vi "GUI_HTT_CTRLv5.vi"() -> ()   [LabVIEW 2020]
uses:
  Shared/GUI_Template/GUI_master/tcp_new_data_event.ctl
  Shared/GUI_Template/GUI_master/tcp new data cluster.ctl
  GUI_TestStand/Fire button.ctl
  <vilib>/Utility/config.llb/Write Key (I32).vi
  <vilib>/Utility/config.llb/Write Key (String).vi
  <vilib>/Platform/browser.llb/Open URL in Default Browser (string).vi
  <vilib>/Utility/config.llb/NI_LVConfig.lvlib
panel:
  out "Opening Time High Value":dbl
  in  "GUIdevice 18":string="HTT-DG645_6_B"
  in  "GUIdevice 17":string="HTT-ManualParameterBool"
  in  "MagSpecGUI 2":bool caption="PicoL GUI"
  out "Delay.Ch C::16":dbl caption="Lamp Timing (680 us is max.)" min=-1.0 max=1.0 format="%#_6e"
  in  "GUIdevice 16":string="HTT-DG645_5Hz"
  in  "AJG Builds":bool caption="PicoB GUI"
  in  "HTW Wiki":bool caption="Google Drive"
  in  "GEECS Website":bool caption="Google Drive"
  in  "HELP":bool caption="Google Drive"
  in  "GUIdevice 15":string="HTT-NewportXPS"
  in  "OK Button":bool
  in  "Date":string="0"
  in  "Create Log":bool caption="LogTable"
  in  "Scan":T1(ring)
  out "standard output":string
  in  "LogEpilog":bool caption="LogTable"
  in  "New day new log":bool=TRUE
  in  "LogTable":bool
  in  "PicoL2":bool caption="PicoL GUI"
  in  "1Wire B GUI":bool caption="PicoL GUI"
  out "fire::12":string="fire" caption="fire"
  in  "Wavelength.Channel0::14":enum16{"248", "355", "532", "800", "2940"}(ring)=enum."532"
  in  "Wavelength.Channel1::14":enum16{"248", "355", "532", "800", "2940"}(ring)=enum."800"
  in  "Wavelength.Channel0::13":enum16{"532", "800"}(ring)=enum."800"
  in  "EnergyRange.Channel0::14":T2(ring)=enum."400mJ"
  in  "EnergyRange.Channel1::14":T2(ring)=enum."400mJ"
  in  "EnergyRange.Channel0::13":T3(ring)=enum."200mJ"
  in  "energy.channel 1::14":dbl caption="Energy Gaia" min=0.0 max=200.0 format="%#_13g"
  out "Energy (J)":dbl
  in  "Multiplicator":dbl=15.3
  in  "GUIdevice 14":string="HTT-Energy-S-G"
  in  "Calibration X":dbl=66.6
  in  "Multiplicator Scatter":dbl=100.0
  out "Energy Scatter (J)":dbl
  out "Energy (J)":dbl
  in  "energy.channel 0::13":dbl caption="Energy Drive" min=0.0 max=10.0 format="%#_13g"
  in  "energy.channel 0::14":dbl caption="Energy Scatter" min=0.0 max=20.0 format="%#_13g"
  in  "GUIdevice 13":string="HTT-Energy-D"
  in  "IR Pt Exp And Comp":bool caption="PicoL GUI"
  in  "Position.Axis 2::10":dbl caption="y/vert." min=-6000.0 max=6000.0
  in  "Position.Axis 3::10":dbl caption="Scatter Mode z" min=-100.0 max=100.0
  in  "Position.Axis 1::10":dbl caption="x/hor." min=-150.0 max=150.0
  in  "Position.Axis 2::11":dbl caption="Translation" min=-50.0 max=50.0
  in  "Position.Axis 3::11":dbl caption="Rotation G1" min=-360.0 max=360.0
  in  "Position.Axis 1::11":dbl caption="Rotation G2" min=-360.0 max=360.0
  in  "Ethernet Powerstrip":bool caption="Google Drive"
  in  "Position.Axis 3::4":dbl caption="z" min=-20.0 max=26.0
  in  "Position.Axis 1::15":dbl caption="Delay Stage" min=-600.0 max=600.0
  in  "FilterWheelB1":bool caption="PicoB GUI"
  in  "Search Log":bool caption="PicoL GUI"
  in  "Experiment \n(if, shadow, topjet)":bool caption="PicoL GUI"
  in  "RemoteDesktop":bool caption="PicoL GUI"
  in  "Experiment \n(e-profile, xrays)":bool caption="PicoL GUI"
  in  "IR TC Pointing (17s)":bool caption="PicoL GUI"
  in  "Scatter Depletion":bool caption="PicoL GUI"
  in  "Scatter IR Amps":bool caption="PicoL GUI"
  in  "Drive TC Pt":bool caption="PicoL GUI"
  in  "Gaia Profiles":bool caption="PicoL GUI"
  in  "Gaia Pointing":bool caption="PicoL GUI"
  in  "IR Exp and Comp":bool caption="PicoL GUI"
  in  "HTT Interactive":bool caption="PicoL GUI"
  in  "GUIdevice 12":string="HTT-DG645"
  in  "Delay.Ch C::12":dbl caption="Delay" min=-0.1 max=2.0 format="%#_6e"
  in  "Delay.Ch D::12":dbl caption="Width" min=-0.1 max=2.0 format="%#_6e"
  in  "Amplitude.Ch CD::12":dbl caption="DG645" min=0.5 max=5.0
  in  "Field::1":dbl caption="B-Field" min=0.0 max=10000.0
  in  "Delay.Ch A::18":dbl caption="Delay" min=0.0 max=1.0 format="%#_6e"
  in  "Delay.Ch B::18":dbl caption="Width" min=0.0 max=1.0 format="%#_6e"
  in  "Amplitude.Ch AB::18":dbl caption="Cam Trig Amp" min=0.5 max=5.0
  in  "1Wire L GUI":bool caption="PicoL GUI"
  in  "Opt. Spectrometer":bool caption="PicoL GUI"
  in  "SingleCamGUI":bool caption="PicoL GUI"
  in  "Exp Editor":bool caption="PicoL GUI"
  in  "DB Editor":bool caption="PicoL GUI"
  in  "Laser Log":bool caption="PicoL GUI"
  in  "LoasisNetDropSchedule":bool caption="PicoL GUI"
  in  "LVStarter":bool caption="PicoL GUI"
  in  "MasterControl":bool caption="PicoL GUI"
  in  "MagSpecGUI":bool caption="PicoL GUI"
  in  "HTT Daily Ops Google Folder":bool caption="Google Drive"
  in  "Depletion Cams":bool caption="PicoL GUI"
  in  "D-L-Cams":bool caption="PicoL GUI"
  in  "Position.Axis 2::5":dbl caption="Mode Out z" min=0.0 max=150.0
  in  "Position.Axis 1::4":dbl caption="Blade" min=-25.0 max=25.0
  in  "Amplitude.Ch CD::18":dbl caption="Trigger Amplitude (V)" min=0.5 max=5.0
  in  "Position.Axis 3::5":dbl caption="Drive Mode In z" min=0.0 max=150.0
  in  "Position.Axis 1::5":dbl caption="Mode Out Wedge" min=0.0 max=25.0
  out "Position.Axis3::2":dbl caption="Rotation G1" min=-180.0 max=180.0 format="%#_13g"
  out "Position.Axis2::2":dbl caption="Rotation G2" min=-180.0 max=180.0 format="%#_13g"
  in  "Position.Axis1::2":dbl caption="Translation" min=-60000.0 max=60000.0 format="%#_13g"
  in  "PicoL":bool caption="PicoL GUI"
  in  "PicoB":bool caption="PicoB GUI"
  in  "AnalogOutput.Channel 0::9":dbl caption="Pressure Ctrl (V)" min=0.0 max=10.0
  in  "Delay.Ch D::18":dbl caption="Opening time (s)" min=0.0 max=100000000000.0 format="%#_6e"
  in  "value1::17":bool caption="Jet Enable"
  in  "value0::17":bool caption="Jet Trigger"
  in  "Position.Axis 3::3":dbl caption="Jet Z" min=0.0 max=25.0
  in  "Position.Axis 2::3":dbl caption="Jet Y" min=11.8 max=25.0
  in  "Position.Axis 1::3":dbl caption="Jet X" min=0.0 max=25.0
  in  "Position.Axis 3::6":dbl caption="Probe delay" min=0.0 max=200.0
  in  "GUIdevice 11":string="HTT-ESP05"
  in  "GUIdevice 8":string="HTT-BNC"
  in  "GUIdevice 6":string="HTT-ESP04"
  in  "GUIdevice 5":string="HTT-ESP03"
  in  "Fire Button":T4=TRUE
  out "error IO 2":errorcluster
  out "fire::10":string
  out "tcp data event":T5
  in  "UDP error message":string
  in  "GUIdevice 7":string="HTT-Pulsar"
  in  "GUIdevice 2":string="HTT-Aerotech"
  in  "GUIdevice 10":string="HTT-ESP06"
  in  "GUIdevice 4":string="HTT-ESP02"
  in  "GUIdevice 1":string="HTT-MagTeslameter-DTM141"
  in  "GUIdevice 3":string="HTT-ESP01"
  in  "GUIdevice 9":string="HTT-HighPressureDAQ"
  in  "Delay.Ch C::18":dbl caption="Jet timing (s)" min=0.0 max=100.0 format="%#_6f"
  in  "stop":bool
  # "Energy"
  # "CAP"
  # "HTT CONTROL CENTER"
  # "Drive"
  # "Gas Jet"
  # "GUI Collection"
  # "Compressor"
  # "Drive Cameras"
  # "Mode Imager"
  # "Probe Delay Line"
  # "Scatter Cameras"
  # "Scatter"
  # "Compressor"
  # "Electronics"
  # "DG645_6_B"
  # "Mode Imager"
  # "Experiment GUIs"
  # "Scatter Delay vs. Drive"
  # "Turning Mirror"
  # "MC Links"
  # "Docu"
  # "Log Maker"
  # "Energy"
  # "yyyy, mm, dd"
  # "Adjustment GUIs"
  # "Drive"
  # "Drive Comp."
  # "Scatter"
  # "Range"
  # "Wavelength"
  # "v0.7   04/16/2021"
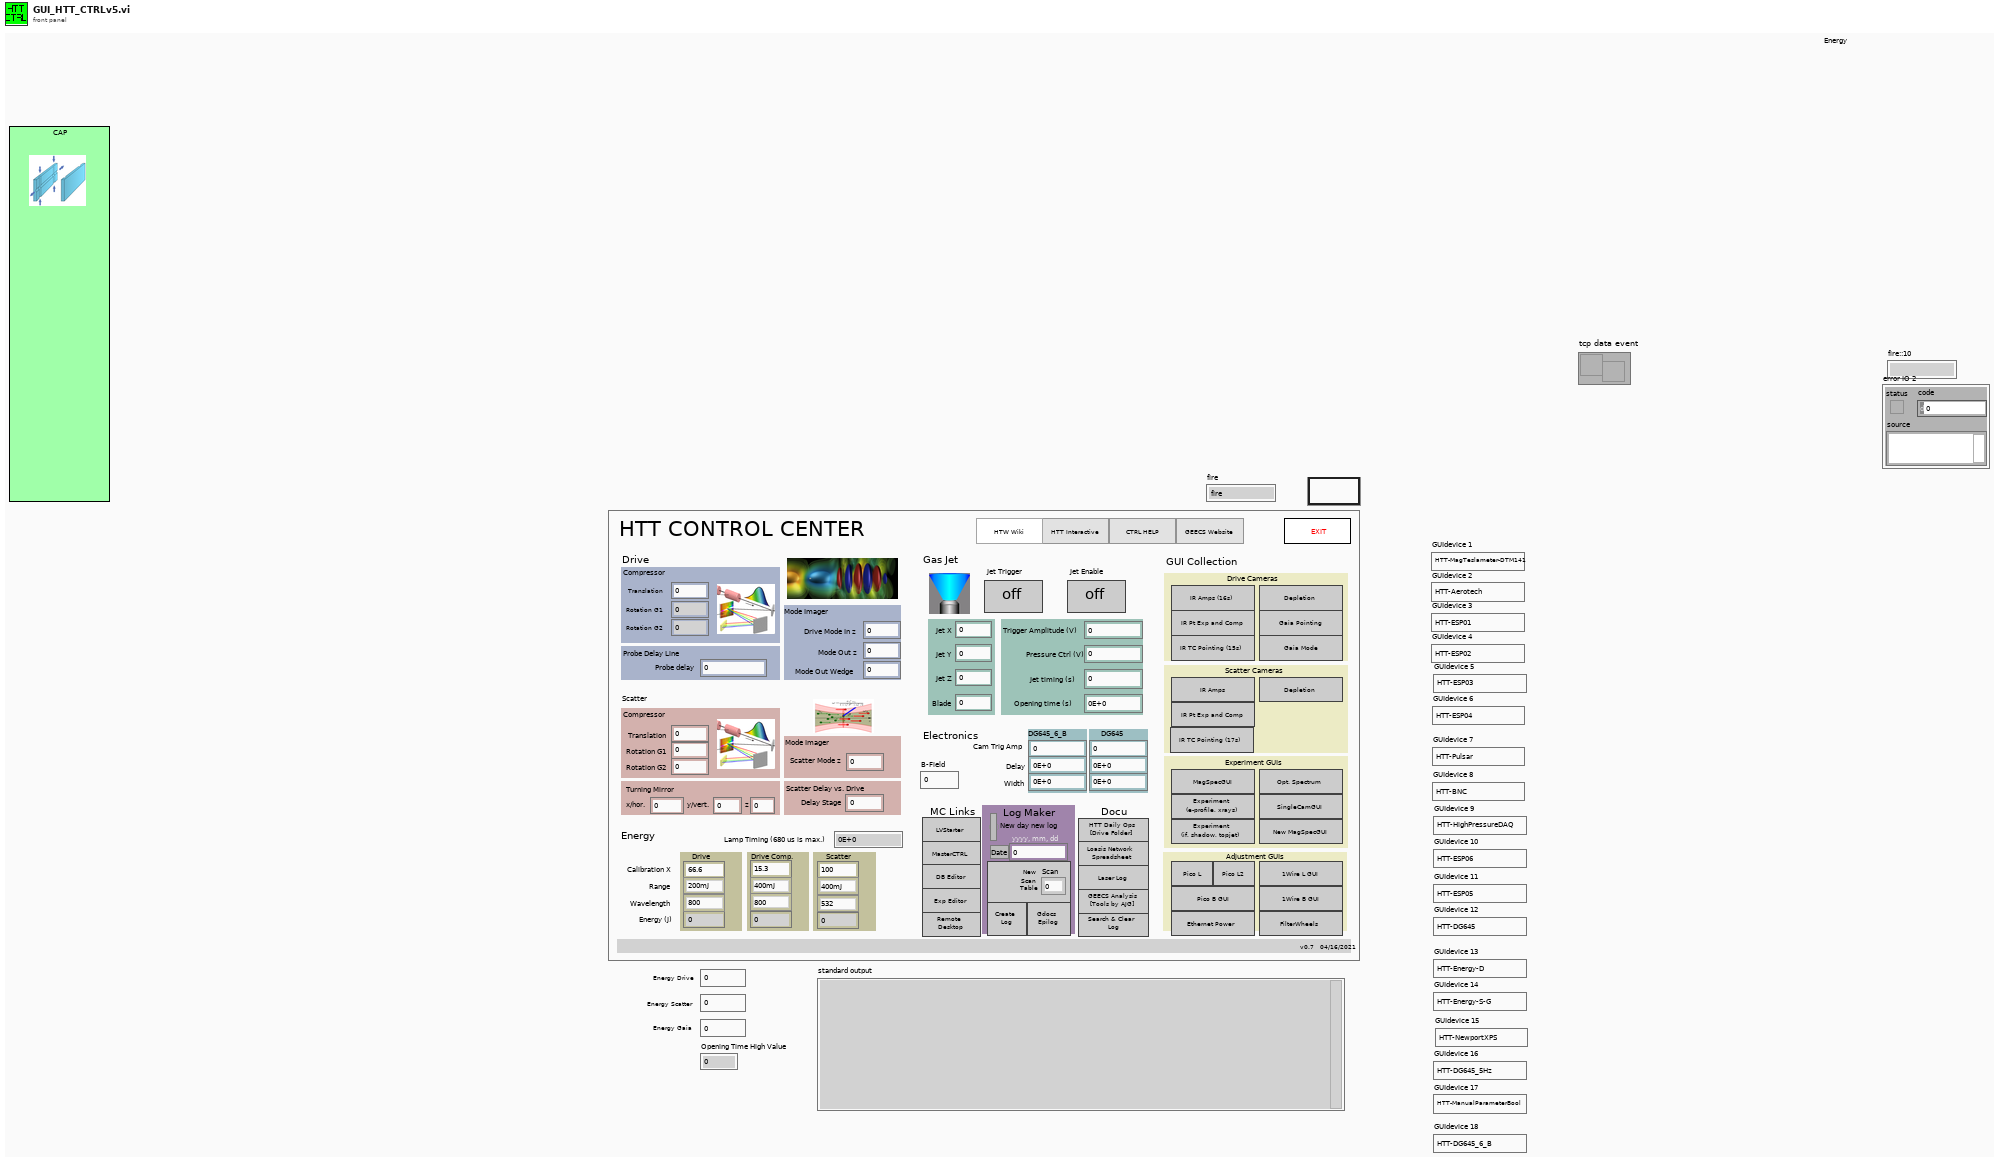
[diagram p1: front panel]
types:
  T1 = enum16{"0", "1", "2", "3", "4", "5", "6", "7", "8", "9", "10", "11", "12", "13", "14", "15", "16", "17", "18", "19", "20", "21", "22", "23", "24", "25", "26", "27", "28", "29", "30", "31", "32", "33", "34", "35", "36", "37", "38", "39", "40", "41", "42", "43", "44", "45", "46", "47", "48", "49", "50", "51", "52", "53", "54", "55", "56", "57", "58", "59", "60", "61", "62", "63", "64", "65", "66", "67", "68", "69", "70", "71", "72", "73", "74", "75", "76", "77", "78", "79", "81", "82", "83", "84", "85", "86", "87", "88", "89", "90", "91", "92", "93", "94", "95", "96", "97", "98", "99", ""}
  T2 = enum16{"4.00mJ", "40.0mJ", "400mJ", "4.00J", "20.00J"}
  T3 = enum16{"2.00mJ", "20.0mJ", "200mJ", "2.00J", "10J"}
  T4 = typedef "Fire button.ctl" = bool
  T5 = typedef "tcp_new_data_event.ctl" = refnum<user-event>
  T6 = typedef "tcp new data cluster.ctl" = cluster{"EventEnum":enum16{"new data", "connection status update"}, "Device name":string}
  T7 = enum32{"invalid app kind", "Development System", "Run Time System", "Student Edition", "Embedded LabVIEW", "Evaluation", "Custom"}
  T8 = enum32{"Invalid", "Standard", "Closed", "Hidden", "Minimized", "Maximized"}
  T9 = cluster{"Core":cluster{"Current VI Reference":refnum<vi>, "Close Panel on Exit?":bool}, "Heater timing offset":dbl, "Discharge timing offset":dbl, "Jet trigger":bool, "Tik1":u32, "Tik2":u32, "Fire Continues Allowed":bool, "Jet enable":bool}
  T10 = typedef "mysql_authentication.ctl" = cluster{"User":string, "Password":string, "Database":string}
  T11 = cluster{"Port":u16, "IP Address":string, "Authentication":T10}
  T12 = typedef "imagedata.ctl" = cluster{"image type":i32, "image depth":i32, "image":u8[], "mask":u8[], "colors":u32[], "Rectangle":cluster{"left":i16, "top":i16, "right":i16, "bottom":i16}}
  T13 = typedef "NI_LVConfig.lvlib/Config Data RefNum.ctl" = refnum<k1>
  T14 = cluster{"Current VI Reference":refnum<vi>, "Close Panel on Exit?":bool}
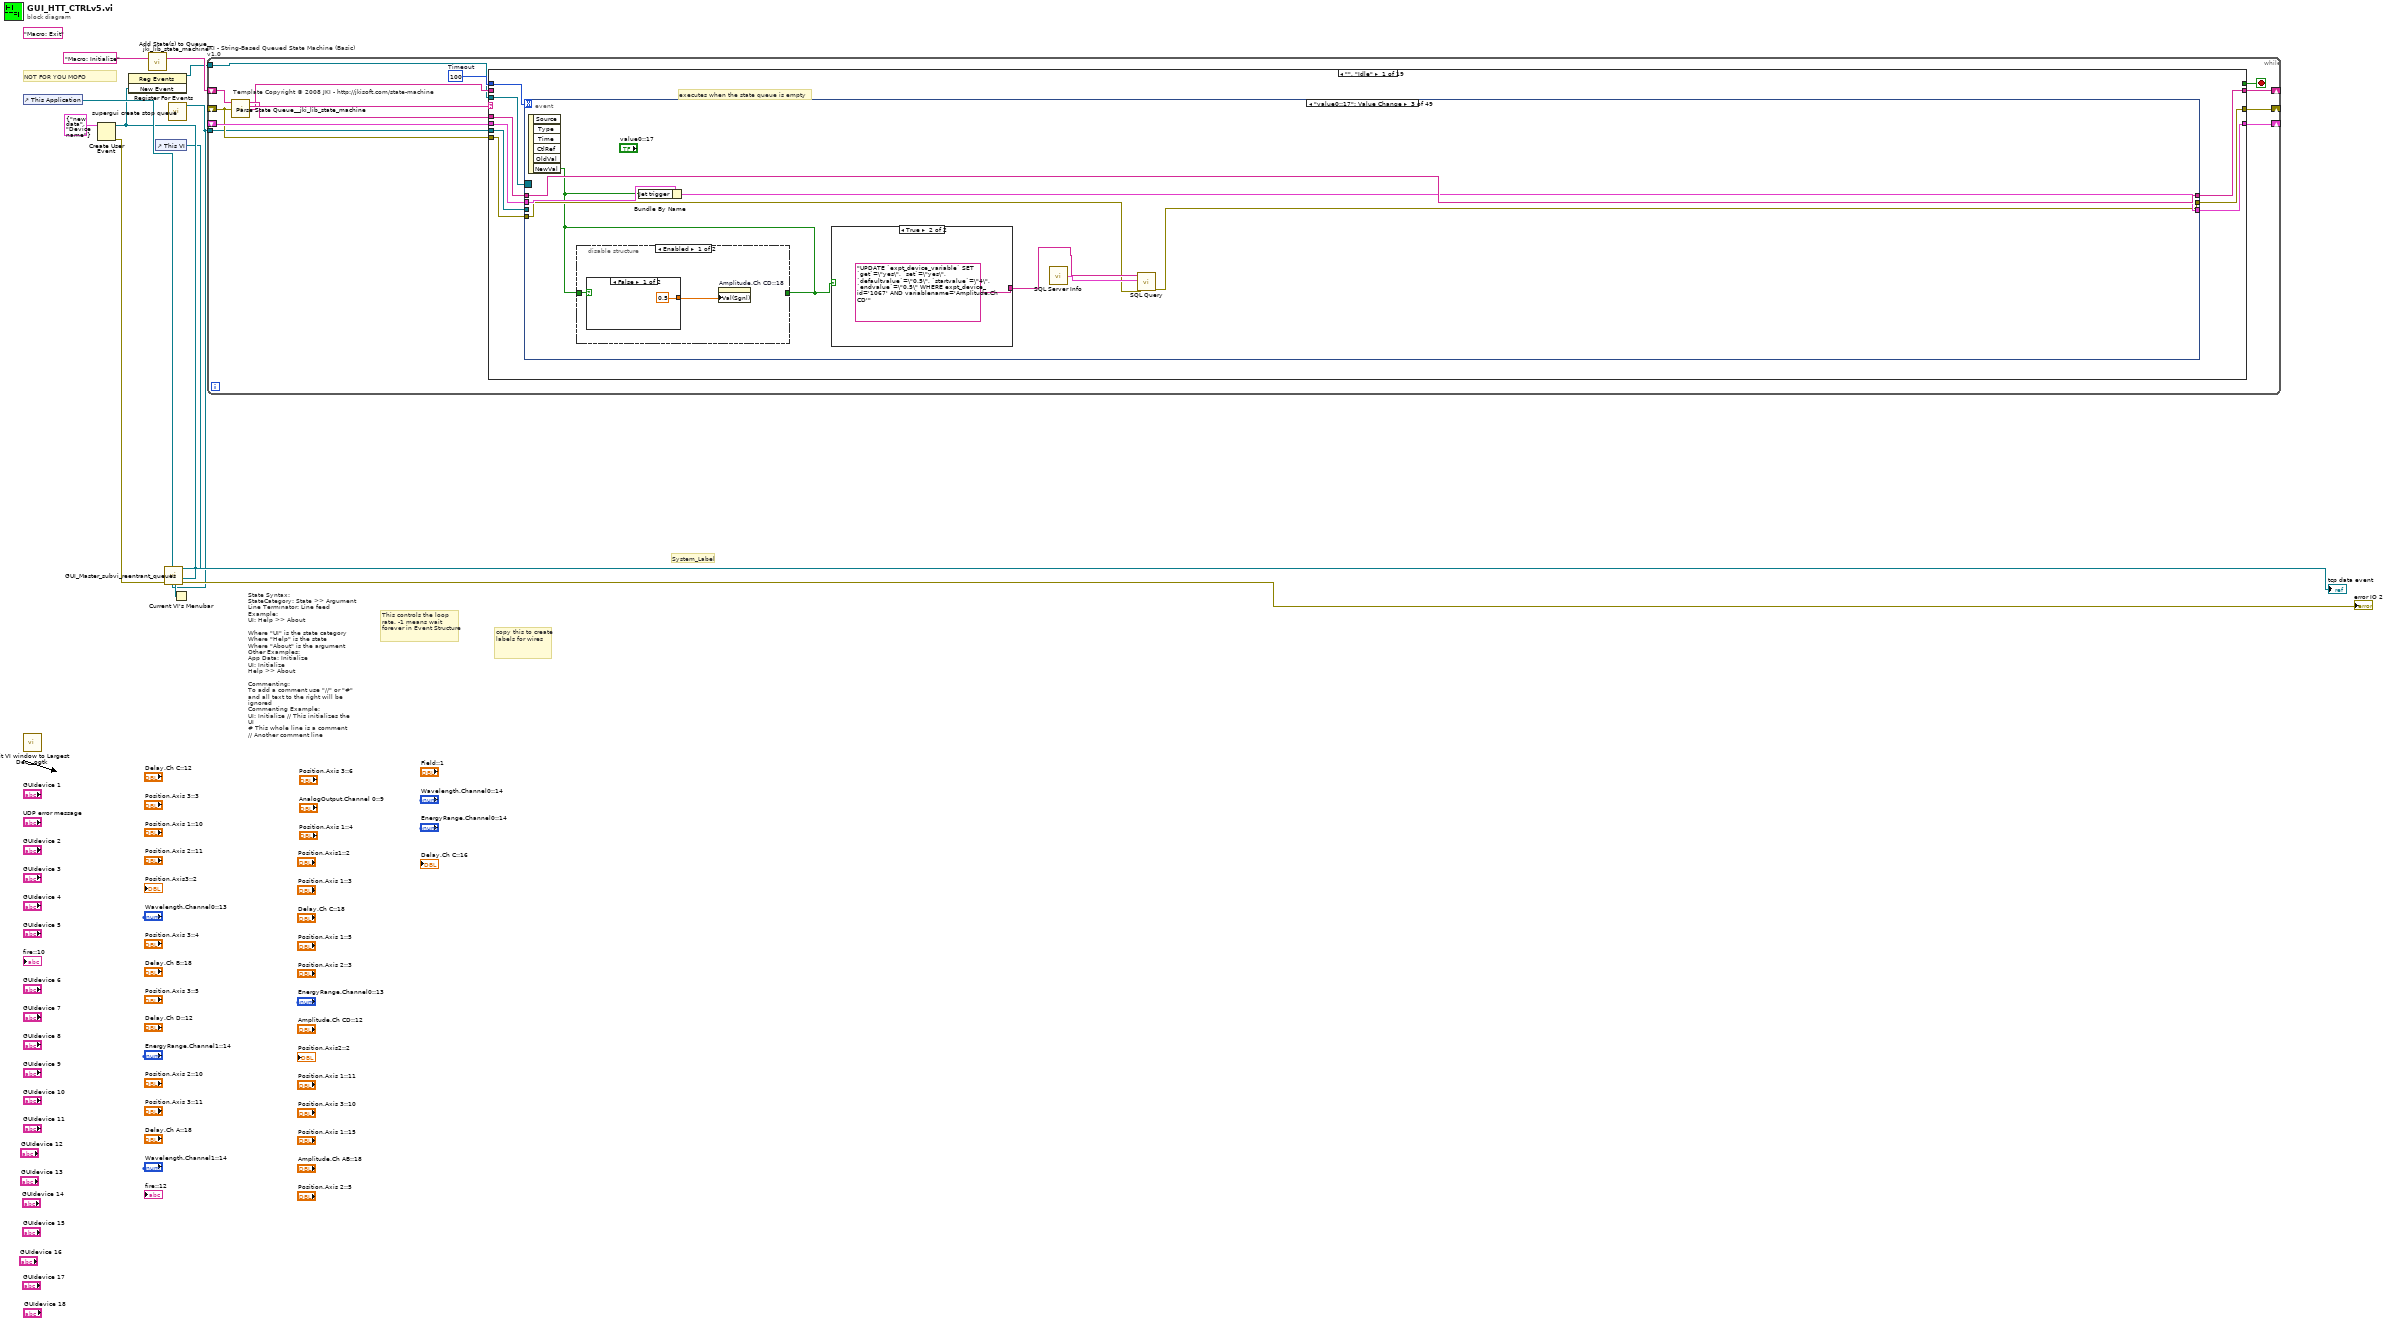
[diagram p0: block diagram]
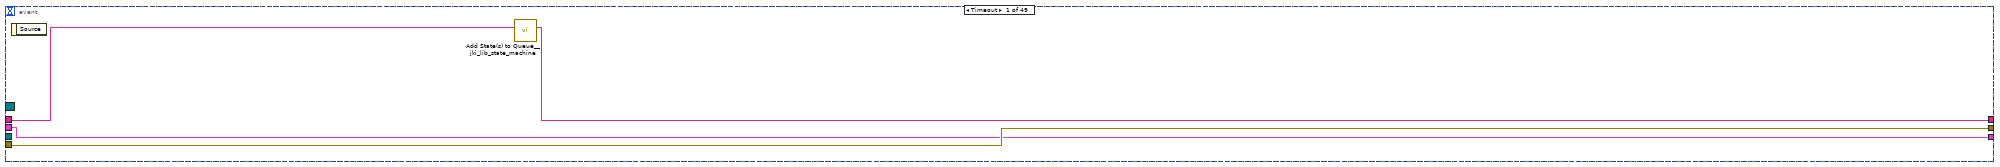
[diagram p2: hidden frame]
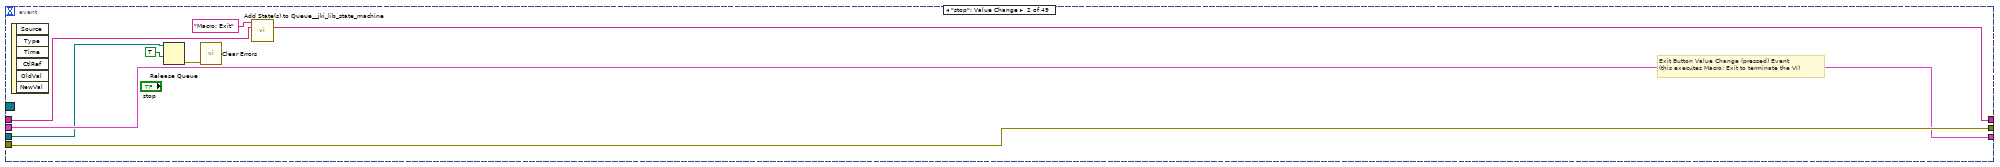
[diagram p3: hidden frame]
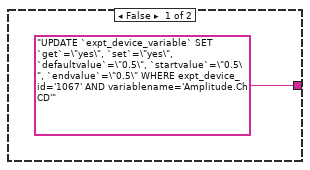
[diagram p4: hidden frame]
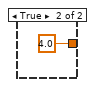
[diagram p5: hidden frame]
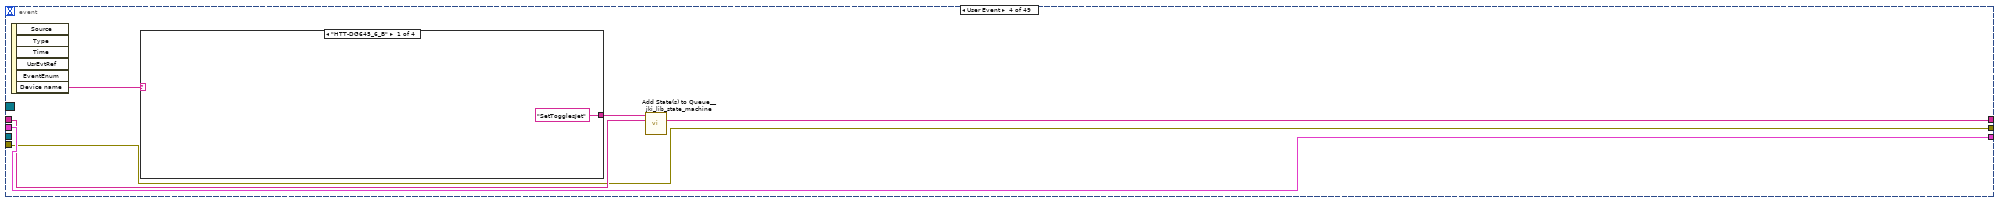
[diagram p7: hidden frame]
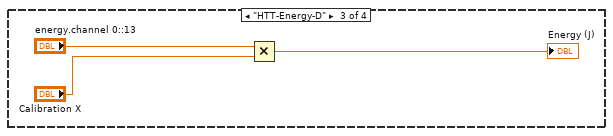
[diagram p9: hidden frame]
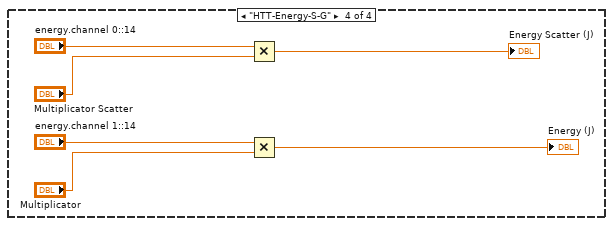
[diagram p10: hidden frame]
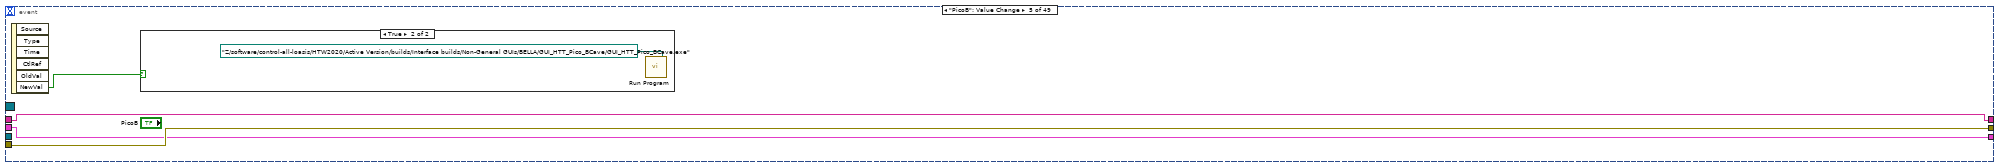
[diagram p11: hidden frame]
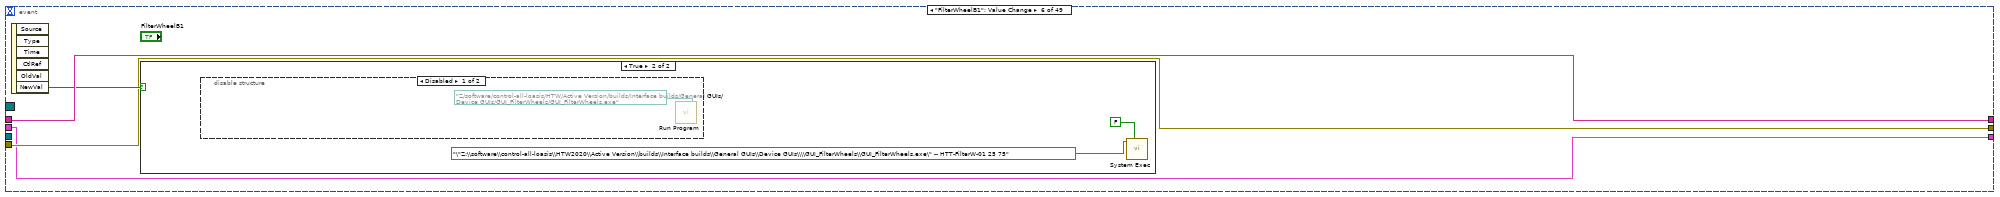
[diagram p13: hidden frame]
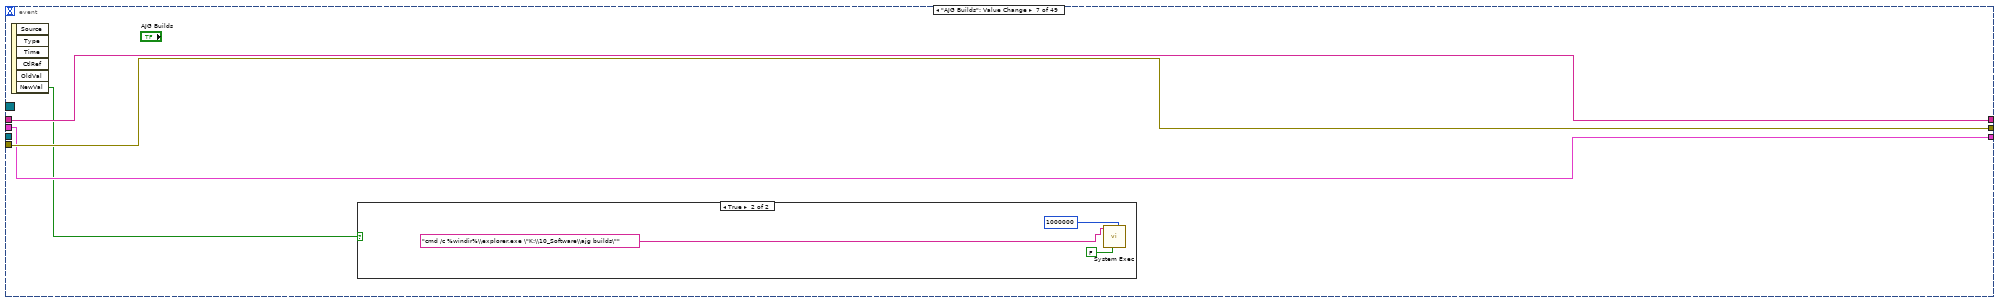
[diagram p16: hidden frame]
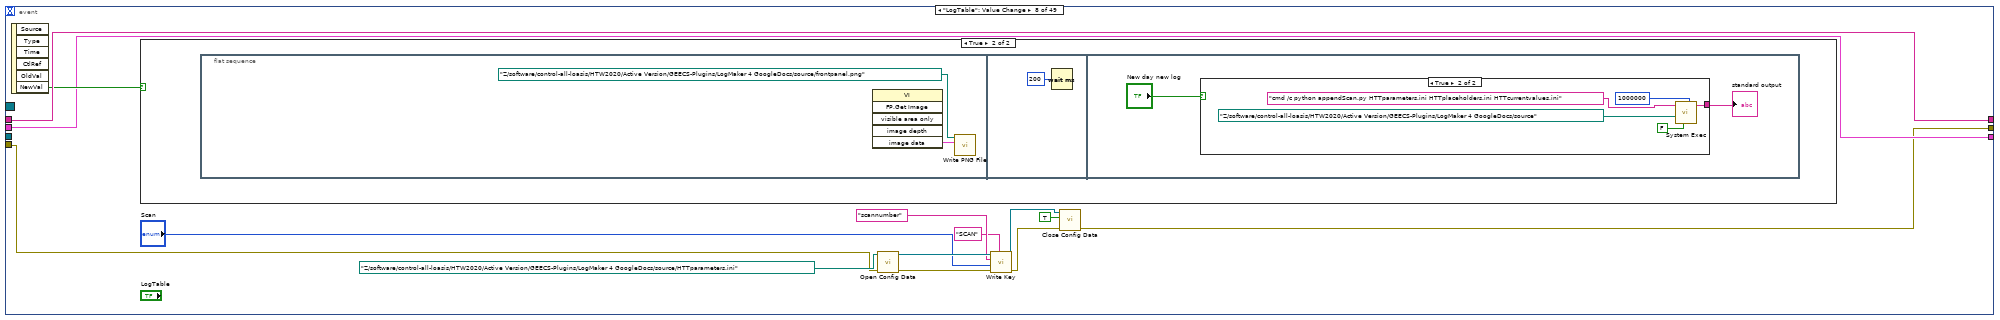
[diagram p18: hidden frame]
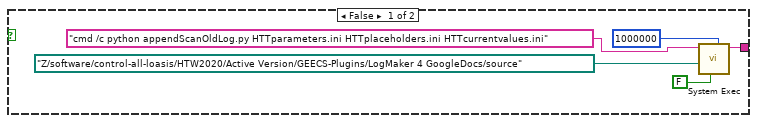
[diagram p20: hidden frame]
diagram:
  (unwired) "Macro: Exit"
  # "State Syntax:\nStateCategory: State >> Argument\nLine Terminator: Line feed\nExample:\nUI: Help >> About\n\nWhere \"UI\" is the state category\nWhere \"Help\" is the state\nWhere \"About\" is the argument\nOther Examples:\nApp Data: Initialize\nUI: Initialize\nHelp >> About\n\nCommenting:\nTo add a comment use \"//\" or \"#\" and all text to the right will be ignored\nCommenting Example:\nUI: Initialize // This initializes the UI\n# This whole line is a comment\n// Another comment line"
  # "copy this to create labels for wires"
  # "This controls the loop rate. -1 means wait forever in Event Structure"
  # "System_Label"
  # "NOT FOR YOU MOFO"
  n1 = control-ref of="This Application"() -> (w11:refnum<vi>)
  n2 = call <userlib>:"Fit VI window to Largest Dec__ogtk.vi"() -> ()  [unwired: 6 in, 2 out]
  n3 = Create User Event(user event datatype=T6 {"EventEnum"=enum."new data", "Device name"="Device name"} ("New Event")) -> (user event=w10:refnum<user-event>, error out=w9:errorcluster)  [unwired: 1 in]
  "tcp data event" <- w10
  n4 = register-events(w10) -> (reference out=w1:refnum<event-registration>)  [unwired: 2 in, 1 out]
  n5 = call <vilib>:"Add State(s) to Queue__jki_lib_state_machine.vi"("State(s) in (\"\")"="Macro: Initialize") -> ("States Out"=w3:string)  [unwired: 14 in]
  n6 = control-ref of="This VI"() -> (w5:refnum<vi>)
  n7 = call "supergui create stop queue.vi"() -> ("STOP Queue out"=w2:refnum<queue>)  [unwired: 11 in]
  n8 = Current VI's Menubar() -> (w7:refnum<k9>)
  n9 = call "GUI_Master_subvi_reentrant_queues.vi"("STOP Queue in"=w2, "This Application"=w11, "error in (no error)"=w9, "tcp data event"=w10, "Caller menu reference"=w7, "Caller VI ref"=w5) -> ("error out"=→"error IO 2":errorcluster)  [unwired: 5 in]
  n10 = while "JKI - String-Based Queued State Machine (Basic) v1.0" {
    shift-right: [w18] -> _
    shift-left: _ -> [w17]
    shift-right: [w20] -> _
    shift-left: _ -> [w15]
    shift-right: [w19] -> _
    shift-left: w3 -> [w21]
    tunnel: w1 -> [w14]
    tunnel: w2 -> [w13]
    stop <- w12 stop-if-true
    w16 = 100  # Timeout
    # "Template Copyright © 2008 JKI - http://jkisoft.com/state-machine"
    n11 = call <vilib>:"Parse State Queue__jki_lib_state_machine.vi"("State Queue"=w21, "Error In (no error)"=w15) -> ("Remaining States"=w23:string, "Current State"=w24:string, "Arguments"=w22:string)  [unwired: 11 in]
    n12 = case shown="\"\", \"Idle\"" w24 {
      selector: w24 -> [_ _ _ w385 _ _ _ _ _ _ _ _ _ _ _ _ _ _ _]
      tunnel: w23 -> [w33 w379 w384 w389 w407 w413 w418 w422 w434 w440 w444 w448 w454 w465 w491 w496 w506 w510 w516]
      tunnel: w22 -> [_ _ _ _ _ _ _ _ _ _ _ _ w449 w459 _ _ _ _ _]
      tunnel: w17 -> [w31 w380 w381 w387 w398 w410 w416 w419 _ w435 w441 w446 w452 w461 w488 w493 w503 w507 w514]
      tunnel: [w30 w378 w382 w391 w404 errorcluster {"status"=FALSE, "code"=0, "source"=""} ("error out") w415 w420 w431 w436 w442 w445 w450 w462 w489 w494 w504 w508 w511] -> w20
      tunnel: w15 -> [w29 w378 w382 w390 w404 w409 w415 w420 w431 w437 w442 w445 w451 w463 w489 w494 w504 w508 w512]
      tunnel: [w32 w379 w383 w388 w406 w412 w417 w421 w433 w439 w443 w447 w453 w464 w490 w495 w505 w509 w515] -> w19
      tunnel: [_ _ _ _ _ _ TRUE _ _ _ _ _ _ _ _ _ _ _ _] -> w12
      tunnel: [w25 w380 w381 w387 w405 w410 w416 w419 w432 w435 w441 w446 w452 w461 w488 w493 w503 w507 w514] -> w18
      tunnel: w16 -> [w28 _ _ _ _ _ _ _ _ _ _ _ _ _ _ _ _ _ _]
      tunnel: w14 -> [w27 _ _ _ _ _ _ _ _ _ _ _ _ _ _ _ _ _ _]
      tunnel: w13 -> [w26 _ _ _ _ _ _ _ _ _ _ _ _ _ _ _ _ _ _]
      frame "", "Idle" {
        # "executes when the state queue is empty"
        n13 = event shown="[2] \"value0::17\": Value Change" {
          selector: w27 -> [_ _ _ _ _ _ _ _ _ _ _ _ _ _ _ _ _ _ _ _ _ _ _ _ _ _ _ _ _ _ _ _ _ _ _ _ _ _ _ _ _ _ _ _ _ _ _ _ _]
          dyn-events: _ -> [_ _ _ _ _ _ _ _ _ _ _ _ _ _ _ _ _ _ _ _ _ _ _ _ _ _ _ _ _ _ _ _ _ _ _ _ _ _ _ _ _ _ _ _ _ _ _ _ _]
          timeout: w28 -> [_ _ _ _ _ _ _ _ _ _ _ _ _ _ _ _ _ _ _ _ _ _ _ _ _ _ _ _ _ _ _ _ _ _ _ _ _ _ _ _ _ _ _ _ _ _ _ _ _]
          tunnel: w33 -> [w37 w45 w53 w63 w79 w84 w91 w108 w128 w144 w152 w160 w165 w170 w175 w180 w185 w190 w195 w200 w205 w210 w215 w220 w225 w230 w235 w240 w245 w250 w255 w260 w265 w270 w275 w280 w285 w290 w295 w300 w305 w310 w315 w320 w325 w334 w349 w355 w365]
          tunnel: [w36 w44 w53 w62 w79 w84 w91 w108 w128 w144 w152 w160 w165 w170 w175 w180 w185 w190 w195 w200 w205 w210 w215 w220 w225 w230 w235 w240 w245 w250 w255 w260 w265 w270 w275 w280 w285 w290 w295 w300 w305 w310 w315 w320 w325 w334 w350 w356 w364] -> w32
          tunnel: w31 -> [w34 w42 w52 w64 w76 w81 w89 w106 w127 w141 w149 w157 w162 w167 w172 w177 w182 w187 w192 w197 w202 w207 w212 w217 w222 w227 w232 w237 w242 w247 w252 w257 w262 w267 w272 w277 w282 w287 w292 w297 w302 w307 w312 w317 w322 w333 w352 w358 w362]
          tunnel: [w35 w43 w47 w61 w77 w82 w90 w95 w125 w142 w150 w158 w163 w168 w173 w178 w183 w188 w193 w198 w203 w208 w213 w218 w223 w228 w233 w238 w243 w248 w253 w258 w263 w268 w273 w278 w283 w288 w293 w298 w303 w308 w313 w318 w323 w327 w351 w357 w363] -> w30
          tunnel: w29 -> [w35 w43 w48 w61 w77 w82 w90 w96 w126 w142 w150 w158 w163 w168 w173 w178 w183 w188 w193 w198 w203 w208 w213 w218 w223 w228 w233 w238 w243 w248 w253 w258 w263 w268 w273 w278 w283 w288 w293 w298 w303 w308 w313 w318 w323 w329 w351 w357 w363]
          tunnel: [w34 w42 w51 w64 w76 w81 w89 w106 w127 w141 w149 w157 w162 w167 w172 w177 w182 w187 w192 w197 w202 w207 w212 w217 w222 w227 w232 w237 w242 w247 w252 w257 w262 w267 w272 w277 w282 w287 w292 w297 w302 w307 w312 w317 w322 w332 w352 w358 w362] -> w25
          tunnel: w26 -> [_ w39 _ _ _ _ _ _ _ _ _ _ _ _ _ _ _ _ _ _ _ _ _ _ _ _ _ _ _ _ _ _ _ _ _ _ _ _ _ _ _ _ _ _ _ _ _ _ _]
          event Timeout {
            n14 = event-data() -> ()  [unwired: 1 in, 1 out]
            n15 = call <vilib>:"Add State(s) to Queue__jki_lib_state_machine.vi"("State(s) in (\"\")"=w37) -> ("States Out"=w36:string)  [unwired: 14 in]
          }
          event "stop": Value Change {
            # "Exit Button Value Change (pressed) Event\n(this executes Macro: Exit to terminate the VI)"
            n16 = event-data() -> ()  [unwired: 1 in, 6 out]
            n17 = Release Queue(queue=w39, force destroy? (F)=TRUE) -> (error out=w40:errorcluster)  [unwired: 1 in, 2 out]
            n18 = call <vilib>:"Clear Errors.vi"("error in (no error)"=w40) -> ()  [unwired: 5 in, 2 out]
            n19 = call <vilib>:"Add State(s) to Queue__jki_lib_state_machine.vi"("State(s) in Front (\"\")"="Macro: Exit", "State(s) in (\"\")"=w45) -> ("States Out"=w44:string)  [unwired: 13 in]
          }
          event "value0::17": Value Change {
            n20 = event-data() -> ("NewVal"=w46:bool)  [unwired: 1 in, 5 out]
            n21 = disable-structure shown="Enabled" {
              disable-tunnel: w46 -> [w57 _]
              disable-tunnel: w46 -> [_ _]
              frame Enabled {
                n22 = case shown="False" w57 {
                  tunnel: [0.5 ("Amplitude.Ch CD::10") 4.0 ("Amplitude.Ch CD::10")] -> w56
                  frame False {
                  }
                  frame True {
                  }
                }
                n23 = property on="Amplitude.Ch CD::18" class="DigNum (strict)"("Val(Sgnl)"=w56) -> ()  [unwired: 2 in, 2 out]
              }
              frame Disabled {
              }
            }
            n24 = Bundle By Name(cluster=w52, "Jet trigger"=w46) -> (w51:T9)
            n25 = case shown="True" w46 {
              tunnel: ["UPDATE `expt_device_variable` SET `get`=\"yes\", `set`=\"yes\", `defaultvalue`=\"0.5\", `startvalue`=\"0.5\", `endvalue`=\"0.5\" WHERE expt_device_id='1067' AND variablename='Amplitude.Ch CD'" ("Query") "UPDATE `expt_device_variable` SET `get`=\"yes\", `set`=\"yes\", `defaultvalue`=\"0.5\", `startvalue`=\"4\", `endvalue`=\"0.5\" WHERE expt_device_id='1067' AND variablename='Amplitude.Ch CD'" ("Query")] -> w49
              frame False {
              }
              frame True {
              }
            }
            n26 = call "SQL Server Info.vi"() -> ("SQL Server Info"=w50:T11)
            n27 = call "SQL Query.vi"("error in (no error)"=w48, "SQL Server Info"=w50, "Query"=w49) -> ("error out"=w47:errorcluster)  [unwired: 7 in, 1 out]
          }
          event User Event {
            n28 = event-data() -> ("Device name"=w65:string)  [unwired: 1 in, 5 out]
            n29 = case shown="\"HTT-DG645_6_B\"" w65 {
              tunnel: ["SetTogglesJet" _ _ _] -> w60
              frame "HTT-DG645_6_B" {
              }
              frame "False", Default {
              }
              frame "HTT-Energy-D" {
                n30 = Multiply(x="energy.channel 0::13", y="Calibration X") -> (x*y=→"Energy (J)":dbl)
              }
              frame "HTT-Energy-S-G" {
                n31 = Multiply(x="energy.channel 0::14", y="Multiplicator Scatter") -> (x*y=→"Energy Scatter (J)":dbl)
                n32 = Multiply(x="energy.channel 1::14", y="Multiplicator") -> (x*y=→"Energy (J)":dbl)
              }
            }
            n33 = call <vilib>:"Add State(s) to Queue__jki_lib_state_machine.vi"("State(s) in Front (\"\")"=w60, "State(s) in (\"\")"=w63) -> ("States Out"=w62:string)  [unwired: 13 in]
          }
          event "PicoB": Value Change {
            n34 = event-data() -> ("NewVal"=w78:bool)  [unwired: 1 in, 5 out]
            n35 = case shown="True" w78 {
              frame False {
              }
              frame True {
                n36 = call "Run Program.vi"("Program Path"=path "Z:/software/control-all-loasis/HTW2020/Active Version/builds/Interface builds/Non-General GUIs/BELLA/GUI_HTT_Pico_BCave/GUI_HTT_Pico_BCave.exe") -> ()  [unwired: 1 in]
              }
            }
          }
          event "FilterWheelB1": Value Change {
            n37 = event-data() -> ("NewVal"=w83:bool)  [unwired: 1 in, 5 out]
            n38 = case shown="True" w83 {
              frame False {
              }
              frame True {
                n39 = disable-structure shown="Disabled" {
                  frame Disabled {
                    n40 = call "Run Program.vi"("Program Path"=path "Z:/software/control-all-loasis/HTW/Active Version/builds/Interface builds/General GUIs/Device GUIs/GUI_FilterWheels/GUI_FilterWheels.exe") -> ()  [unwired: 1 in]
                  }
                  frame Enabled {
                  }
                }
                n41 = call <vilib>:"System Exec.vi"("wait until completion? (T)"=FALSE, "command line"="\"Z:\\software\\control-all-loasis\\HTW2020\\Active Version\\builds\\Interface builds\\General GUIs\\Device GUIs\\\\GUI_FilterWheels\\GUI_FilterWheels.exe\" -- HTT-FilterW-01 25 75") -> ()  [unwired: 6 in, 4 out]
              }
            }
          }
          event "AJG Builds": Value Change {
            n42 = event-data() -> ("NewVal"=w88:bool)  [unwired: 1 in, 5 out]
            n43 = case shown="True" w88 {
              frame False {
              }
              frame True {
                n44 = call <vilib>:"System Exec.vi"("expected output size  (4096)"=u32 1000000, "run minimized? (F)"=FALSE, "command line"="cmd /c %windir%\\explorer.exe \"K:\\10_Software\\ajg builds\"") -> ()  [unwired: 5 in, 4 out]
              }
            }
          }
          event "LogTable": Value Change {
            n45 = event-data() -> ("NewVal"=w107:bool)  [unwired: 1 in, 5 out]
            n46 = case shown="True" w107 {
              frame False {
              }
              frame True {
                n47 = flat-sequence {
                  frame #0 {
                    n48 = invoke class="VI" method="FP.Get Image"() -> ("image data"=w110:T12)  [unwired: 6 in, 5 out]
                    n49 = call <vilib>:"Write PNG File.vi"("image data"=w110, "path to PNG file"=path "Z:/software/control-all-loasis/HTW2020/Active Version/GEECS-Plugins/LogMaker 4 GoogleDocs/source/frontpanel.png" ("report file path")) -> ()  [unwired: 8 in, 2 out]
                  }
                  frame #1 {
                    n50 = Wait (ms)(milliseconds to wait=u32 200 ("millisecond timer value")) -> ()  [unwired: 1 out]
                  }
                  frame #2 {
                    n51 = case shown="True" "New day new log" {
                      tunnel: [w114 w119] -> w112
                      frame False {
                        n52 = call <vilib>:"System Exec.vi"("expected output size  (4096)"=u32 1000000, "run minimized? (F)"=FALSE, "working directory"=path "Z:/software/control-all-loasis/HTW2020/Active Version/GEECS-Plugins/LogMaker 4 GoogleDocs/source", "command line"="cmd /c python appendScanOldLog.py HTTparameters.ini HTTplaceholders.ini HTTcurrentvalues.ini") -> ("standard output"=w114:string)  [unwired: 4 in, 3 out]
                      }
                      frame True {
                        n53 = call <vilib>:"System Exec.vi"("expected output size  (4096)"=u32 1000000, "run minimized? (F)"=FALSE, "working directory"=path "Z:/software/control-all-loasis/HTW2020/Active Version/GEECS-Plugins/LogMaker 4 GoogleDocs/source", "command line"="cmd /c python appendScan.py HTTparameters.ini HTTplaceholders.ini HTTcurrentvalues.ini") -> ("standard output"=w119:string)  [unwired: 4 in, 3 out]
                      }
                    }
                    "standard output" <- w112
                  }
                }
              }
            }
            n54 = call <vilib>:"Open Config Data.vi"("error in (no error)"=w96, "configuration file path"=path "Z:/software/control-all-loasis/HTW2020/Active Version/GEECS-Plugins/LogMaker 4 GoogleDocs/source/HTTparameters.ini") -> ("error out"=w102:errorcluster, "refnum"=w104:T13)  [unwired: 7 in, 1 out]
            n55 = call-poly <vilib>:"Write Key.vi"("section"="SCAN", "error in (no error)"=w102, "value"="Scan", "key"="scannumber", "refnum"=w104) -> ("error out"=w101:errorcluster, "refnum out"=w103:T13)  [unwired: 4 in, 1 out]
            n56 = call <vilib>:"Close Config Data.vi"("error in (no error)"=w101, "write file if changed (T)"=TRUE, "refnum"=w103) -> ("error out"=w95:errorcluster)  [unwired: 7 in, 1 out]
          }
          event "OK Button": Value Change {
            n57 = event-data() -> ("NewVal"=w124:bool)  [unwired: 1 in, 5 out]
            n58 = case shown="True" w124 {
              tunnel: w126 -> [w129 w132]
              tunnel: [w129 w131] -> w125
              frame False {
              }
              frame True {
                n59 = call <vilib>:"Open Config Data.vi"("error in (no error)"=w132, "configuration file path"=path "Z:/software/control-all-loasis/HTW2020/Active Version/GEECS-Plugins/LogMaker 4 GoogleDocs/source/HTTparameters.ini") -> ("error out"=w137:errorcluster, "refnum"=w139:T13)  [unwired: 7 in, 1 out]
                n60 = call-poly <vilib>:"Write Key.vi"("section"="DATE", "error in (no error)"=w137, "value"="Date", "key"="specificdate", "refnum"=w139) -> ("error out"=w136:errorcluster, "refnum out"=w138:T13)  [unwired: 4 in, 1 out]
                n61 = call <vilib>:"Close Config Data.vi"("error in (no error)"=w136, "write file if changed (T)"=TRUE, "refnum"=w138) -> ("error out"=w131:errorcluster)  [unwired: 7 in, 1 out]
              }
            }
          }
          event "LogEpilog": Value Change {
            n62 = event-data() -> ("NewVal"=w143:bool)  [unwired: 1 in, 5 out]
            n63 = case shown="True" w143 {
              frame False {
              }
              frame True {
                n64 = call <vilib>:"System Exec.vi"("expected output size  (4096)"=u32 1000000, "run minimized? (F)"=FALSE, "working directory"=path "Z:/software/control-all-loasis/HTW2020/Active Version/GEECS-Plugins/LogMaker 4 GoogleDocs/source", "command line"="cmd /c python appendEpilog.py HTTparameters.ini HTTplaceholders.ini HTTcurrentvalues.ini") -> ()  [unwired: 4 in, 4 out]
              }
            }
          }
          event "Create Log": Value Change {
            n65 = event-data() -> ("NewVal"=w151:bool)  [unwired: 1 in, 5 out]
            n66 = case shown="True" w151 {
              frame False {
              }
              frame True {
                n67 = call <vilib>:"System Exec.vi"("expected output size  (4096)"=u32 1000000, "run minimized? (F)"=FALSE, "working directory"=path "Z:/software/control-all-loasis/HTW2020/Active Version/GEECS-Plugins/LogMaker 4 GoogleDocs/source", "command line"="cmd /c python createGdoc.py HTTparameters.ini HTTplaceholders.ini HTTcurrentvalues.ini") -> ()  [unwired: 4 in, 4 out]
              }
            }
          }
          event "PicoL": Value Change {
            n68 = event-data() -> ("NewVal"=w159:bool)  [unwired: 1 in, 5 out]
            n69 = case shown="True" w159 {
              frame False {
              }
              frame True {
                n70 = call "Run Program.vi"("Program Path"=path "Z:/software/control-all-loasis/HTW2020/Active Version/builds/Interface builds/Non-General GUIs/BELLA/GUI_HTT_Pico_LCave/GUI_HTT_Pico_LCave.exe") -> ()  [unwired: 1 in]
              }
            }
          }
          event "PicoL2": Value Change {
            n71 = event-data() -> ("NewVal"=w164:bool)  [unwired: 1 in, 5 out]
            n72 = case shown="True" w164 {
              frame False {
              }
              frame True {
                n73 = call "Run Program.vi"("Program Path"=path "Z:/software/control-all-loasis/HTW2020/Active Version/builds/Interface builds/Non-General GUIs/BELLA/GUI_HTT_Pico_LCave2/GUI_HTT_Pico_LCave2.exe") -> ()  [unwired: 1 in]
              }
            }
          }
          event "D-L-Cams": Value Change {
            n74 = event-data() -> ("NewVal"=w169:bool)  [unwired: 1 in, 5 out]
            n75 = case shown="True" w169 {
              frame False {
              }
              frame True {
                n76 = call "Run Program.vi"("Program Path"=path "Z:/software/control-all-loasis/HTW2020/Active Version/builds/Interface builds/Non-General GUIs/BELLA/GUI_HTT_MultiCamDriveAmp/GUI_HTT_MultiCamsDriveAmp.exe") -> ()  [unwired: 1 in]
              }
            }
          }
          event "Depletion Cams": Value Change {
            n77 = event-data() -> ("NewVal"=w174:bool)  [unwired: 1 in, 5 out]
            n78 = case shown="True" w174 {
              frame False {
              }
              frame True {
                n79 = call "Run Program.vi"("Program Path"=path "Z:/software/control-all-loasis/HTW2020/Active Version/builds/Interface builds/Non-General GUIs/BELLA/GUI_HTT_MultiCamDriveAmp/GUI_HTT_MultiCamsDriveDepletion.exe") -> ()  [unwired: 1 in]
              }
            }
          }
          event "Gaia Profiles": Value Change {
            n80 = event-data() -> ("NewVal"=w179:bool)  [unwired: 1 in, 5 out]
            n81 = case shown="True" w179 {
              frame False {
              }
              frame True {
                n82 = call "Run Program.vi"("Program Path"=path "Z:/software/control-all-loasis/HTW2020/Active Version/builds/Interface builds/Non-General GUIs/BELLA/GUI_HTT_MultiCamDriveAmp/GUI_HTT_MultiCamsDriveGaiaProfile.exe") -> ()  [unwired: 1 in]
              }
            }
          }
          event "Drive TC Pt": Value Change {
            n83 = event-data() -> ("NewVal"=w184:bool)  [unwired: 1 in, 5 out]
            n84 = case shown="True" w184 {
              frame False {
              }
              frame True {
                n85 = call "Run Program.vi"("Program Path"=path "Z:/software/control-all-loasis/HTW2020/Active Version/builds/Interface builds/Non-General GUIs/BELLA/GUI_HTT_MultiCamDriveAmp/GUI_HTT_MultiCamsDriveTCPointing.exe") -> ()  [unwired: 1 in]
              }
            }
          }
          event "Scatter IR Amps": Value Change {
            n86 = event-data() -> ("NewVal"=w189:bool)  [unwired: 1 in, 5 out]
            n87 = case shown="True" w189 {
              frame False {
              }
              frame True {
                n88 = call "Run Program.vi"("Program Path"=path "Z:/software/control-all-loasis/HTW2020/Active Version/builds/Interface builds/Non-General GUIs/BELLA/GUI_HTT_MultiCamDriveAmp/GUI_HTT_MultiCamsScatterAmp.exe") -> ()  [unwired: 1 in]
              }
            }
          }
          event "Scatter Depletion": Value Change {
            n89 = event-data() -> ("NewVal"=w194:bool)  [unwired: 1 in, 5 out]
            n90 = case shown="True" w194 {
              frame False {
              }
              frame True {
                n91 = call "Run Program.vi"("Program Path"=path "Z:/software/control-all-loasis/HTW2020/Active Version/builds/Interface builds/Non-General GUIs/BELLA/GUI_HTT_MultiCamDriveAmp/GUI_HTT_MultiCamsScatterDepletion.exe") -> ()  [unwired: 1 in]
              }
            }
          }
          event "IR Exp and Comp": Value Change {
            n92 = event-data() -> ("NewVal"=w199:bool)  [unwired: 1 in, 5 out]
            n93 = case shown="True" w199 {
              frame False {
              }
              frame True {
                n94 = call "Run Program.vi"("Program Path"=path "Z:/software/control-all-loasis/HTW2020/Active Version/builds/Interface builds/Non-General GUIs/BELLA/GUI_HTT_MultiCamDriveAmp/GUI_HTT_MultiCamsDriveExpAndComp.exe") -> ()  [unwired: 1 in]
              }
            }
          }
          event "Gaia Pointing": Value Change {
            n95 = event-data() -> ("NewVal"=w204:bool)  [unwired: 1 in, 5 out]
            n96 = case shown="True" w204 {
              frame False {
              }
              frame True {
                n97 = call "Run Program.vi"("Program Path"=path "Z:/software/control-all-loasis/HTW2020/Active Version/builds/Interface builds/Non-General GUIs/BELLA/GUI_HTT_MultiCamDriveAmp/GUI_HTT_MultiCamsDriveGaiaPointing.exe") -> ()  [unwired: 1 in]
              }
            }
          }
          event "1Wire L GUI": Value Change {
            n98 = event-data() -> ("NewVal"=w209:bool)  [unwired: 1 in, 5 out]
            n99 = case shown="True" w209 {
              frame False {
              }
              frame True {
                n100 = call "Run Program.vi"("Program Path"=path "Z:/software/control-all-loasis/HTW/Active Version/builds/Interface builds/Non-General GUIs/BELLA/GUI_HTT_1Wire/GUI_HTT_1Wire.exe") -> ()  [unwired: 1 in]
              }
            }
          }
          event "1Wire B GUI": Value Change {
            n101 = event-data() -> ("NewVal"=w214:bool)  [unwired: 1 in, 5 out]
            n102 = case shown="True" w214 {
              frame False {
              }
              frame True {
                n103 = call "Run Program.vi"("Program Path"=path "Z:/software/control-all-loasis/HTW2020/Active Version/builds/Interface builds/Non-General GUIs/BELLA/GUI_HTT_1Wire_BCave/GUI_HTT_1Wire_BCave.exe") -> ()  [unwired: 1 in]
              }
            }
          }
          event "MagSpecGUI": Value Change {
            n104 = event-data() -> ("NewVal"=w219:bool)  [unwired: 1 in, 5 out]
            n105 = case shown="True" w219 {
              frame False {
              }
              frame True {
                n106 = call "Run Program.vi"("Program Path"=path "Z:/software/control-all-loasis/HTW2020/Active Version/builds/Interface builds/Non-General GUIs/BELLA/GUI_HTT_MultiCamDriveAmp/GUI_HTT_MultiCamsDriveMagSpec.exe") -> ()  [unwired: 1 in]
              }
            }
          }
          event "MagSpecGUI 2": Value Change {
            n107 = event-data() -> ("NewVal"=w224:bool)  [unwired: 1 in, 5 out]
            n108 = case shown="True" w224 {
              frame False {
              }
              frame True {
                n109 = call "Run Program.vi"("Program Path"=path "Z:/software/control-all-loasis/HTW2020/Active Version/builds/Interface builds/General GUIs/Device GUIs/GUI_Cameras/GUI_Cameras.exe -- HTT-C14_1_new_espec 25 75") -> ()  [unwired: 1 in]
              }
            }
          }
          event "IR TC Pointing (17s)": Value Change {
            n110 = event-data() -> ("NewVal"=w229:bool)  [unwired: 1 in, 5 out]
            n111 = case shown="True" w229 {
              frame False {
              }
              frame True {
                n112 = call "Run Program.vi"("Program Path"=path "Z:/software/control-all-loasis/HTW2020/Active Version/builds/Interface builds/Non-General GUIs/BELLA/GUI_HTT_MultiCamDriveAmp/GUI_HTT_MultiCamsScatterTCPointing.exe") -> ()  [unwired: 1 in]
              }
            }
          }
          event "IR Pt Exp And Comp": Value Change {
            n113 = event-data() -> ("NewVal"=w234:bool)  [unwired: 1 in, 5 out]
            n114 = case shown="True" w234 {
              frame False {
              }
              frame True {
                n115 = call "Run Program.vi"("Program Path"=path "Z:/software/control-all-loasis/HTW2020/Active Version/builds/Interface builds/Non-General GUIs/BELLA/GUI_HTT_MultiCamDriveAmp/GUI_HTT_MultiCamsScatterExpAndComp.exe") -> ()  [unwired: 1 in]
              }
            }
          }
          event "Experiment \n(e-profile, xrays)": Value Change {
            n116 = event-data() -> ("NewVal"=w239:bool)  [unwired: 1 in, 5 out]
            n117 = case shown="True" w239 {
              frame False {
              }
              frame True {
                n118 = call "Run Program.vi"("Program Path"=path "Z:/software/control-all-loasis/HTW2020/Active Version/builds/Interface builds/Non-General GUIs/BELLA/GUI_HTT_MultiCamDriveAmp/GUI_HTT_MultiCamsDriveExperiment1.exe") -> ()  [unwired: 1 in]
              }
            }
          }
          event "Experiment \n(if, shadow, topjet)": Value Change {
            n119 = event-data() -> ("NewVal"=w244:bool)  [unwired: 1 in, 5 out]
            n120 = case shown="True" w244 {
              frame False {
              }
              frame True {
                n121 = call "Run Program.vi"("Program Path"=path "Z:/software/control-all-loasis/HTW2020/Active Version/builds/Interface builds/Non-General GUIs/BELLA/GUI_HTT_MultiCamDriveAmp/GUI_HTT_MultiCamsDriveExperiment2.exe") -> ()  [unwired: 1 in]
              }
            }
          }
          event "MasterControl": Value Change {
            n122 = event-data() -> ("NewVal"=w249:bool)  [unwired: 1 in, 5 out]
            n123 = case shown="True" w249 {
              frame False {
              }
              frame True {
                n124 = call "Run Program.vi"("Program Path"=path "Z:/software/control-all-loasis/HTW2020/Active Version/builds/Interface builds/General GUIs/MC/Master Control/Master Control.exe") -> ()  [unwired: 1 in]
              }
            }
          }
          event "LVStarter": Value Change {
            n125 = event-data() -> ("NewVal"=w254:bool)  [unwired: 1 in, 5 out]
            n126 = case shown="True" w254 {
              frame False {
              }
              frame True {
                n127 = call "Run Program.vi"("Program Path"=path "Z:/software/control-all-loasis/HTW2020/Active Version/builds/Interface builds/General GUIs/MC/LVstarter/LVstarter.exe") -> ()  [unwired: 1 in]
              }
            }
          }
          event "LoasisNetDropSchedule": Value Change {
            n128 = event-data() -> ("NewVal"=w259:bool)  [unwired: 1 in, 5 out]
            n129 = case shown="True" w259 {
              frame False {
              }
              frame True {
                n130 = call-poly <vilib>:"Open URL in Default Browser.vi"("URL"="https://docs.google.com/spreadsheets/d/1jCB4RWAsyhhLTDJV5kG2lLZ6BYZGIF6lGWV0o1NQmIw/edit#gid=446136478") -> ()  [unwired: 5 in, 2 out]
              }
            }
          }
          event "Laser Log": Value Change {
            n131 = event-data() -> ("NewVal"=w264:bool)  [unwired: 1 in, 5 out]
            n132 = case shown="True" w264 {
              frame False {
              }
              frame True {
                n133 = call-poly <vilib>:"Open URL in Default Browser.vi"("URL"="https://docs.google.com/spreadsheets/d/16XvNmISrrBuveoI843fEshmnkqsdwVJN6yzR7b6LCqo/edit#gid=0") -> ()  [unwired: 5 in, 2 out]
              }
            }
          }
          event "DB Editor": Value Change {
            n134 = event-data() -> ("NewVal"=w269:bool)  [unwired: 1 in, 5 out]
            n135 = case shown="True" w269 {
              frame False {
              }
              frame True {
                n136 = call "Run Program.vi"("Program Path"=path "Z:/software/control-all-loasis/HTW2020/Active Version/builds/Interface builds/General GUIs/Database editor/Database editor.exe") -> ()  [unwired: 1 in]
              }
            }
          }
          event "Exp Editor": Value Change {
            n137 = event-data() -> ("NewVal"=w274:bool)  [unwired: 1 in, 5 out]
            n138 = case shown="True" w274 {
              frame False {
              }
              frame True {
                n139 = call "Run Program.vi"("Program Path"=path "Z:/software/control-all-loasis/HTW2020/Active Version/builds/Interface builds/General GUIs/Database editor/Expt_Devices_GUI_Datagridview.exe") -> ()  [unwired: 1 in]
              }
            }
          }
          event "SingleCamGUI": Value Change {
            n140 = event-data() -> ("NewVal"=w279:bool)  [unwired: 1 in, 5 out]
            n141 = case shown="True" w279 {
              frame False {
              }
              frame True {
                n142 = call "Run Program.vi"("Program Path"=path "Z:/software/control-all-loasis/HTW2020/Active Version/builds/Interface builds/General GUIs/Device GUIs/GUI_Cameras/GUI_Cameras.exe") -> ()  [unwired: 1 in]
              }
            }
          }
          event "Opt. Spectrometer": Value Change {
            n143 = event-data() -> ("NewVal"=w284:bool)  [unwired: 1 in, 5 out]
            n144 = case shown="True" w284 {
              frame False {
              }
              frame True {
                n145 = call "Run Program.vi"("Program Path"=path "Z:/software/control-all-loasis/HTW2020/Active Version/builds/Interface builds/Non-General GUIs/BELLA/GUI_HTT_HamamatsuSpec/GUI_HTT_HamamatsuSpec.exe") -> ()  [unwired: 1 in]
              }
            }
          }
          event "RemoteDesktop": Value Change {
            n146 = event-data() -> ("NewVal"=w289:bool)  [unwired: 1 in, 5 out]
            n147 = case shown="True" w289 {
              frame False {
              }
              frame True {
                n148 = call "Run Program.vi"("Program Path"=path "C:/Windows/System32/mstsc.exe") -> ()  [unwired: 1 in]
              }
            }
          }
          event "HTT Daily Ops Google Folder": Value Change {
            n149 = event-data() -> ("NewVal"=w294:bool)  [unwired: 1 in, 5 out]
            n150 = case shown="True" w294 {
              frame False {
              }
              frame True {
                # "HTT daily ops"
                n151 = call-poly <vilib>:"Open URL in Default Browser.vi"("URL"="https://drive.google.com/drive/folders/0B6BJlLNDz1MaOC10bXdFbHFBQ00?usp=sharing") -> ()  [unwired: 5 in, 2 out]
              }
            }
          }
          event "HELP": Value Change {
            n152 = event-data() -> ("NewVal"=w299:bool)  [unwired: 1 in, 5 out]
            n153 = case shown="True" w299 {
              frame False {
              }
              frame True {
                # "HTT daily ops"
                n154 = call-poly <vilib>:"Open URL in Default Browser.vi"("URL"="https://sites.google.com/a/lbl.gov/htw-wiki/how-to-guides/htt-control-center-help/") -> ()  [unwired: 5 in, 2 out]
              }
            }
          }
          event "GEECS Website": Value Change {
            n155 = event-data() -> ("NewVal"=w304:bool)  [unwired: 1 in, 5 out]
            n156 = case shown="True" w304 {
              frame False {
              }
              frame True {
                # "HTT daily ops"
                n157 = call-poly <vilib>:"Open URL in Default Browser.vi"("URL"="https://sites.google.com/a/lbl.gov/geecs/bella?authuser=0") -> ()  [unwired: 5 in, 2 out]
              }
            }
          }
          event "HTW Wiki": Value Change {
            n158 = event-data() -> ("NewVal"=w309:bool)  [unwired: 1 in, 5 out]
            n159 = case shown="True" w309 {
              frame False {
              }
              frame True {
                n160 = call-poly <vilib>:"Open URL in Default Browser.vi"("URL"="https://sites.google.com/a/lbl.gov/htw-wiki/HTW-projects?authuser=0") -> ()  [unwired: 5 in, 2 out]
              }
            }
          }
          event "Ethernet Powerstrip": Value Change {
            n161 = event-data() -> ("NewVal"=w314:bool)  [unwired: 1 in, 5 out]
            n162 = case shown="True" w314 {
              frame False {
              }
              frame True {
                # "Ethernet Powerstrip"
                n163 = call-poly <vilib>:"Open URL in Default Browser.vi"("URL"="http://192.168.6.208/outlet.html") -> ()  [unwired: 5 in, 2 out]
              }
            }
          }
          event "HTT Interactive": Value Change {
            n164 = event-data() -> ("NewVal"=w319:bool)  [unwired: 1 in, 5 out]
            n165 = case shown="True" w319 {
              frame False {
              }
              frame True {
                n166 = call-poly <vilib>:"Open URL in Default Browser.vi"("URL"="https://docs.google.com/presentation/d/1vde03GLRziloe-kxBmiBfXX4-hwSL2uU9dDMmq9JgxY/edit?usp=sharing") -> ()  [unwired: 5 in, 2 out]
              }
            }
          }
          event "Search Log": Value Change {
            n167 = event-data() -> ("NewVal"=w324:bool)  [unwired: 1 in, 5 out]
            n168 = case shown="True" w324 {
              frame False {
              }
              frame True {
                n169 = call-poly <vilib>:"Open URL in Default Browser.vi"("URL"="https://docs.google.com/spreadsheets/d/1wR7To7WJHrQNP-2Id8ScCGPPim0LYwsaw_KNOLmAjJY/edit?usp=sharing") -> ()  [unwired: 5 in, 2 out]
              }
            }
          }
          event "value1::17": Value Change {
            n170 = event-data() -> ("NewVal"=w328:bool)  [unwired: 1 in, 5 out]
            n171 = Bundle By Name(cluster=w333, "Jet enable"=w328) -> (w332:T9)
            n172 = disable-structure shown="Enabled" {
              disable-tunnel: w328 -> [w344 _]
              disable-tunnel: w328 -> [_ _]
              frame Enabled {
                n173 = case shown="True" w344 {
                  tunnel: [0.0 ("opening Time") w346] -> w343
                  frame False {
                  }
                  frame True {
                    n174 = local read "Opening Time High Value"() -> (w346:dbl)
                  }
                }
                n175 = property on="Delay.Ch D::18" class="DigNum (strict)"("Val(Sgnl)"=w343) -> ()  [unwired: 2 in, 2 out]
              }
              frame Disabled {
              }
            }
            n176 = case shown="True" w328 {
              tunnel: ["UPDATE `expt_device_variable` SET `get`=\"yes\", `set`=\"yes\", `defaultvalue`=\"0\", `startvalue`=\"0\", `endvalue`=\"0\" WHERE expt_device_id='1067' AND variablename='Delay.Ch D'" ("Query") w337] -> w330
              frame False {
              }
              frame True {
                n177 = local read "Opening Time High Value"() -> (w336:dbl)
                n178 = Number To Fractional String(number=w336, precision (6)=i16 4) -> (F-format string=w340:string)  [unwired: 2 in]
                n179 = Search and Replace String(replace all?=TRUE ("replace all? (F)"), input string="UPDATE `expt_device_variable` SET `get`=\"yes\", `set`=\"yes\", `defaultvalue`=\"0\", `startvalue`=\"xxx\", `endvalue`=\"0\" WHERE expt_device_id='1067' AND variablename='Delay.Ch D'" ("Query"), search string="xxx", replace string=w340) -> (result string=w337:string)  [unwired: 4 in, 3 out]
              }
            }
            n180 = call "SQL Server Info.vi"() -> ("SQL Server Info"=w331:T11)
            n181 = call "SQL Query.vi"("error in (no error)"=w329, "SQL Server Info"=w331, "Query"=w330) -> ("error out"=w327:errorcluster)  [unwired: 7 in, 1 out]
          }
          event Value Change {
            n182 = event-data() -> ()  [unwired: 1 in, 6 out]
            n183 = property on="fire::12" class="Str"("Val(Sgnl)"="fire>>force" ("Value (Signaling)")) -> ()  [unwired: 2 in, 2 out]
            n184 = call <vilib>:"Add State(s) to Queue__jki_lib_state_machine.vi"("State(s) in Front (\"\")"="Action: Fire" ("State(s) in Front (\"\")"), "State(s) in (\"\")"=w349) -> ("States Out"=w350:string)  [unwired: 13 in]
          }
          event "Delay.Ch D::18": Value Change {
            n185 = event-data() -> ("NewVal"=w353:dbl)  [unwired: 1 in, 5 out]
            n186 = Greater Than 0?(x=w353) -> (x > 0?=w354:bool)
            n187 = call <vilib>:"Add State(s) to Queue__jki_lib_state_machine.vi"("State(s) in (\"\")"=w355) -> ("States Out"=w356:string)  [unwired: 14 in]
            n188 = case shown="True" w354 {
              tunnel: w353 -> [_ w359]
              frame False {
              }
              frame True {
                "Opening Time High Value" <- w359
              }
            }
          }
          event Panel Close? {
            # "Discard the event because we'll close the front panel ourselves in Macro: Exit"
            # "Close Panel button (pressed) Event\n(this executes Macro: Exit to terminate the VI)"
            n189 = event-data() -> ()  [unwired: 1 in, 1 out]
            n190 = call <vilib>:"Add State(s) to Queue__jki_lib_state_machine.vi"("State(s) in Front (\"\")"="Macro: Exit", "State(s) in (\"\")"=w365) -> ("States Out"=w364:string)  [unwired: 13 in]
            n191 = event-data("Discard?"=TRUE) -> ()  [unwired: 1 in, 1 out]
          }
        }
      }
      frame "SetTogglesJet" {
        n192 = Greater?(x="Delay.Ch D::18", y=0.0001) -> (0:w367:bool)
        n193 = Greater?(x="Amplitude.Ch CD::18", y=2.5) -> (0:w375:bool)
        n194 = Select(t=TRUE, s=w367, f=FALSE) -> (s? t:f=w366:bool)
        n195 = Select(t=TRUE, s=w375, f=FALSE) -> (s? t:f=w372:bool)
        n196 = local write "value1::17"(w366) -> ()
        n197 = local write "value0::17"(w372) -> ()
      }
      frame "---------- Core ----------" {
        # "Do not put any code in this frame.\n(it is a separator no-op)"
        n198 = call <vilib>:"Add State(s) to Queue__jki_lib_state_machine.vi"("State(s) in (\"\")"=w384) -> ("States Out"=w383:string)  [unwired: 14 in]
      }
      frame Default {
        w394 = 42 items=["No error", "Argument error", "Memory is full", "Out of zone", "End of file", "File already open", "Generic file I/O error", "File not found", "File permission error", "Disk is full", "Duplicate path", "Too many files open", "System feature not enabled", "Resource file not found", "Cannot add resource", "Resource not found", "Image not found", "Image memory error", "Pen does not exist", "Config type invalid", "Config token not found", "Config parse error", "Config memory error", "Bad external code format", "Bad external code offset", "External code not present", "Null window", "Destroy window error", "Null menu", "Print aborted", "Bad print record", "Print driver error", "Windows error during printing", "Memory error during printing", "Print dialog error", "Generic print error", "Invalid device refnum", "Device not found", "Device parameter error", "Device unit error", "Cannot open device", "Device call aborted", "Generic error", "Cancelled by user", "Object ID too low", "Object ID too high", "Object not in heap", "Unknown heap", "Unknown object (invalid DefProc)", "Unknown object (DefProc not in table)", "Message out of range", "Invalid (null) method", "Unknown message", "Manager call not supported", "Bad address", "Network operation in progress", "Network operation timed out", "Connection is busy", "Network attribute not supported", "Network error", "Address in use", "System out of memory", "Connection aborted", "Connection refused", "Not connected", "Already connected", "Connection closed", "Initialization error (interapplication manager)", "Bad occurrence", "Wait on unbound occurrence handler", "Occurrence queue overflow", "Datalog type conflict", "Unused", "Unrecognized type (interapplication manager)", "Memory corrupt", "Failed to make temporary DLL", "Old CIN version", "Drag socket not found", "Failed to load drop-object", "Failed to register OLE object", "Failed to release OLE object", "Format specifier type mismatch", "Unknown format specifier", "Too few format specifiers", "Too many format specifiers", "Scan failed", "Newer CIN version", "Error converting to variant", "Runtime menu error", "Password tampered", "Variant attribute not found", "Incompatible variant data type", "Event data is not available", "Event Store is not present", "Occurrence is not found", "Event Queue is not created", "Event info is not available", "Refnum passed is NULL", "Error retrieving Class GUID", "Error retrieving CoClass GUID", "Error retrieving TypeLib GUID.", "Bad built application magic bytes.", "Specific driver is different from the specific driver associated with the Logical Name.", "There is no session opened to the class driver.", "Max Error", "MAX - Error with config objects", "MAX - Error loading configuration", "MAX - Group not supported"]
        # "Current State"
        # "Do not delete, rename, or modify this frame.\n(this is used to capture unhandled states and typos)"
        # "Handle mistyped state name (developer tool)"
        n199 = Format Into String(format string="Software Exception: Unhandled State \"%s\"." ("message"), error in=w390, w385) -> (resulting string=w393:string, error out=w392:errorcluster)  [unwired: 1 in]
        n200 = call <vilib>:"Error Cluster From Error Code.vi"("show call chain? (False)"=TRUE, "error in (no error)"=w392, "error message (\"\")"=w393, "error code (0)"=w394) -> ("error out"=w391:errorcluster)  [unwired: 5 in]
        n201 = call <vilib>:"Add State(s) to Queue__jki_lib_state_machine.vi"("State(s) in (\"\")"=w389) -> ("States Out"=w388:string)  [unwired: 14 in]
      }
      frame "Initialize Core Data" {
        # "Do not delete, rename, or modify this frame.\n(this is used to determine panel behavior on exit)"
        # "originally closed?"
        # "exe?"
        # "If panel starts closed or is an EXE, then close it when we exit"
        n202 = property class="VI"() -> ("Front Panel.Open"=w403:bool)  [unwired: 2 in, 2 out]
        n203 = Not(x=w403) -> (.not. x?=w400:bool)
        n204 = property class="App"() -> ("App.Kind"=w402:T7)  [unwired: 2 in, 2 out]
        n205 = Equal?(x=w402, y=T7."Run Time System" ("Application:Kind")) -> (x = y?=w399:bool)
        n206 = control-ref of="Current VI Reference"() -> (w396:refnum<vi>)
        n207 = Or(x=w400, y=w399) -> (x .or. y?=w397:bool)
        n208 = Bundle By Name(cluster=w398, "Core.Current VI Reference"=w396, "Core.Close Panel on Exit?"=w397) -> (w405:T9)
        n209 = call <vilib>:"Add State(s) to Queue__jki_lib_state_machine.vi"("State(s) in (\"\")"=w407) -> ("States Out"=w406:string)  [unwired: 14 in]
      }
      frame "Error Handler" {
        # "Unhandled Error -- Display it"
        # "Handle any errors here.\nYou can also output any states to clean-up after errors occur"
        # "Clear error"
        n210 = call <vilib>:"General Error Handler.vi"("error in (no error)"=w409) -> ()  [unwired: 10 in, 5 out]
        n211 = call <vilib>:"Add State(s) to Queue__jki_lib_state_machine.vi"("State(s) in Front (\"\")"="/* Post Error States", "State(s) in (\"\")"=w413) -> ("States Out"=w412:string)  [unwired: 13 in]
      }
      frame "Exit" {
        # "Do not put any code in this frame.\n(No errors that occur here will be handled.)"
        n212 = call <vilib>:"Add State(s) to Queue__jki_lib_state_machine.vi"("State(s) in (\"\")"=w418) -> ("States Out"=w417:string)  [unwired: 14 in]
      }
      frame "---------- Data ----------" {
        # "Do not put any code in this frame.\n(It is a separator no-op. You can make a copy of this frame to create a new Data frame)"
        n213 = call <vilib>:"Add State(s) to Queue__jki_lib_state_machine.vi"("State(s) in (\"\")"=w422) -> ("States Out"=w421:string)  [unwired: 14 in]
      }
      frame "Data: Initialize" {
        w423 = FALSE  # Jet enable
        w424 = FALSE  # Fire Continues Allowed
        w426 = u32 0  # Tik1
        w425 = u32 0  # Tik2
        w427 = FALSE  # Jet trigger
        w428 = 0.0  # Discharge timing offset
        w429 = 0.0  # Heater timing offset
        w430 = T14 {"Current VI Reference"=refnum, "Close Panel on Exit?"=FALSE}  # Core
        # "do not delete - used by framework"
        # "Expand Bundle to add new data elements to shift register data."
        # "Add new data here."
        # "Data names and types of shift register data are defined by this bundle."
        # "Initialize the shift-register data, here.\n(data names are defined by what you wire into the bundle function)"
        n214 = call <vilib>:"Add State(s) to Queue__jki_lib_state_machine.vi"("State(s) in (\"\")"=w434) -> ("States Out"=w433:string)  [unwired: 14 in]
        n215 = Bundle("Core"=w430, "Heater timing offset"=w429, "Discharge timing offset"=w428, "Jet trigger"=w427, "Tik1"=w426, "Tik2"=w425, "Fire Continues Allowed"=w424, "Jet enable"=w423) -> (w432:T9)  [unwired: 1 in]
      }
      frame "Data: Cleanup" {
        # "Cleanup any data and references, here.\n(this is called automatically, by the Macro: Exit)"
        n216 = Unbundle By Name(w435) -> ("Core.Current VI Reference"=w438:refnum<vi>)
        n217 = Close Reference(reference=w438, error in (no error)=w437) -> (error out=w436:errorcluster)
        n218 = call <vilib>:"Add State(s) to Queue__jki_lib_state_machine.vi"("State(s) in (\"\")"=w440) -> ("States Out"=w439:string)  [unwired: 14 in]
      }
      frame "---------- UI ----------" {
        # "Do not put any code in this frame.\n(It is a separator no-op. You can make a copy of this frame to create a new UI frame)"
        n219 = call <vilib>:"Add State(s) to Queue__jki_lib_state_machine.vi"("State(s) in (\"\")"=w444) -> ("States Out"=w443:string)  [unwired: 14 in]
      }
      frame "UI: Initialize" {
        # "Initialize the User Interface, here.\n(this is called automatically, by the Macro: Init)"
        n220 = call <vilib>:"Add State(s) to Queue__jki_lib_state_machine.vi"("State(s) in (\"\")"=w448) -> ("States Out"=w447:string)  [unwired: 14 in]
      }
      frame "UI: Cursor Set" {
        # "Argument"
        # "Set and Unset Cursor Busy.\n(Usage: \"UI: Cursor Set >> Busy|Idle\")"
        n221 = case shown="\"Idle\", Default" w449 {
          tunnel: w451 -> [w456 w458]
          tunnel: [w455 w457] -> w450
          frame "Idle", Default {
            n222 = call <vilib>:"Unset Busy.vi"("error in (no error)"=w456) -> ("error out"=w455:errorcluster)  [unwired: 10 in]
          }
          frame "Busy" {
            n223 = call <vilib>:"Set Busy.vi"("error in (no error)"=w458) -> ("error out"=w457:errorcluster)  [unwired: 9 in, 1 out]
          }
        }
        n224 = call <vilib>:"Add State(s) to Queue__jki_lib_state_machine.vi"("State(s) in (\"\")"=w454) -> ("States Out"=w453:string)  [unwired: 14 in]
      }
      frame "UI: Front Panel State" {
        # "Argument"
        # "Set Front Panel Open or Closed\n(Usage: \"UI: Front Panel State >> Open|Close\")"
        n225 = Unbundle By Name(w461) -> ("Core.Current VI Reference"=w460:refnum<vi>)
        n226 = case shown="\"Close\"" w459 {
          tunnel: w463 -> [w469 w482]
          tunnel: [w471 w483] -> w462
          tunnel: w460 -> [w470 w480]
          frame "Open", Default {
            n227 = property class="VI"(reference=w470, error in=w469) -> (reference out=w467:refnum<vi>, error out=w468:errorcluster, "Front Panel.Open"=w466:bool)
            n228 = case shown="False" w466 {
              tunnel: [w474 w477] -> w471
              tunnel: w468 -> [w473 w477]
              tunnel: w467 -> [w472 _]
              frame False {
                n229 = invoke class="VI" method="FP.Open"(reference=w472, error in=w473, "Activate"=TRUE, "State"=T8."Standard") -> (error out=w474:errorcluster)  [unwired: 1 in, 4 out]
              }
              frame True {
              }
            }
          }
          frame "Close" {
            n230 = property class="VI"(reference=w480, error in=w482) -> (reference out=w479:refnum<vi>, error out=w481:errorcluster, "Front Panel.Open"=w478:bool)
            n231 = case shown="True" w478 {
              tunnel: [w484 w487] -> w483
              tunnel: w481 -> [w484 w486]
              tunnel: w479 -> [_ w485]
              frame False {
              }
              frame True {
                n232 = invoke class="VI" method="FP.Close"(reference=w485, error in=w486) -> (error out=w487:errorcluster)  [unwired: 1 in, 2 out]
              }
            }
          }
        }
        n233 = call <vilib>:"Add State(s) to Queue__jki_lib_state_machine.vi"("State(s) in (\"\")"=w465) -> ("States Out"=w464:string)  [unwired: 14 in]
      }
      frame "---------- Macro ----------" {
        # "Do not put any code in this frame.\n(It is a separator no-op. You can make a copy of this frame to create a new Macro frame)"
        n234 = call <vilib>:"Add State(s) to Queue__jki_lib_state_machine.vi"("State(s) in (\"\")"=w491) -> ("States Out"=w490:string)  [unwired: 14 in]
      }
      frame "Macro: Initialize" {
        w492 = "Data: Initialize\nInitialize Core Data\nUI: Initialize\nUI: Front Panel State >> Open"  # Data: Initialize Initialize Core Data UI: Initialize UI: Front Panel State >> Open
        # "Initialization Macro\n(This is called once, when the VI starts)"
        n235 = call <vilib>:"Add State(s) to Queue__jki_lib_state_machine.vi"("State(s) in Front (\"\")"=w492, "State(s) in (\"\")"=w496) -> ("States Out"=w495:string)  [unwired: 13 in]
      }
      frame "Macro: Exit" {
        # "Exit Macro\n(This is called once, when the VI exits)"
        n236 = Unbundle By Name(w503) -> ("Core.Close Panel on Exit?"=w502:bool)
        n237 = Select(t="UI: Front Panel State >> Close", s=w502, f="") -> (s? t:f=w499:string)
        n238 = call <vilib>:"Add State(s) to Queue__jki_lib_state_machine.vi"("State(s) in (\"\")"=w499, "State(s) at Back (\"\")"="Data: Cleanup\nExit") -> ("States Out"=w497:string)  [unwired: 13 in]
        n239 = call <vilib>:"Add State(s) to Queue__jki_lib_state_machine.vi"("State(s) in Front (\"\")"=w497, "State(s) in (\"\")"=w506) -> ("States Out"=w505:string)  [unwired: 13 in]
      }
      frame "---------- New Category ----------" {
        # "Template Separator\n(You can make a copy of, or modify, this frame)"
        n240 = call <vilib>:"Add State(s) to Queue__jki_lib_state_machine.vi"("State(s) in (\"\")"=w510) -> ("States Out"=w509:string)  [unwired: 14 in]
      }
      frame "Action: Fire" {
        # "Your code here.\n(You can make a copy of, or modify, this frame)"
        n241 = property on="fire::10" class="Str"(error in=w512, "Val(Sgnl)"="fire>>force" ("Value (Signaling)")) -> (error out=w511:errorcluster)  [unwired: 1 in, 1 out]
        n242 = call <vilib>:"Add State(s) to Queue__jki_lib_state_machine.vi"("State(s) in (\"\")"=w516) -> ("States Out"=w515:string)  [unwired: 14 in]
      }
    }
  }
